vi "create_black_screen.vi"() -> (1 "img_black_screen":T1(plugin-control))   [LabVIEW 2011]
uses:
  global_vars.vi
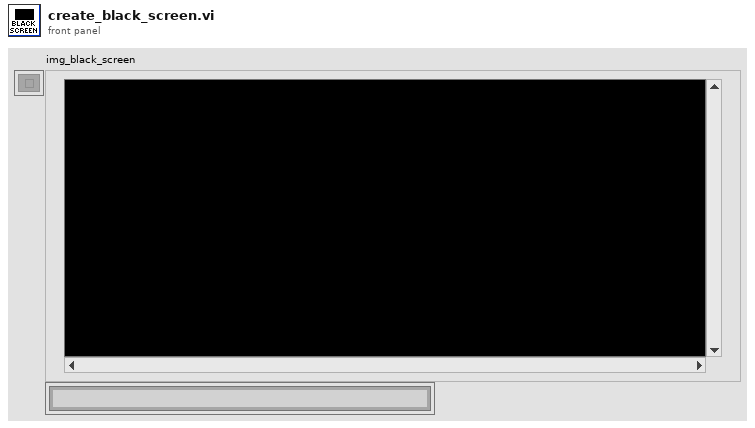
[diagram p1: front panel]
types:
  T1 = typedef "IMAQ Image.ctl" = refnum<image>
  T2 = typedef "Image Type" = u32
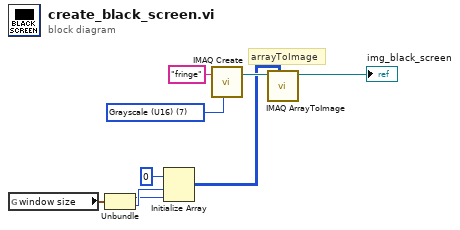
[diagram p0: block diagram]
diagram:
  w5 = T2 7 items=["Grayscale (U8)", "Grayscale (I16)", "Grayscale (SGL)", "Complex (CSG)", "RGB (U32)", "HSL (U32)", "RGB (U64)", "Grayscale (U16)"] ("Image Type")
  # "arrayToImage"
  n1 = global read "global_vars.vi" "window size"() -> (w9:cluster{"x Width(Px)":i32, "y height(Px)":i32})
  n2 = Unbundle(w9) -> ("x Width(Px)"=w3:i32, "y height(Px)"=w4:i32)
  n3 = Initialize Array(u16 0 ("element"), w4, w3) -> (w1:u16[][])
  n4 = call "IMAQ Create"("Image Name"="fringe", "Image Type"=w5) -> ("New Image"=w6:T1)  [unwired: 2 in, 2 out]
  n5 = call "IMAQ ArrayToImage"("Image Pixels (U16)"=w1, "Image"=w6) -> ("Image Out"=→"img_black_screen":T1)  [unwired: 8 in, 1 out]
